vi "arranque.vi"   [LabVIEW 2016]
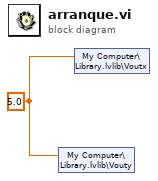
[diagram p0: block diagram]
diagram:
  w1 = 5.0
  n1 = shared-variable "My Computer\\Library.lvlib\\Vouty"(w1) -> ()  [unwired: 1 in, 1 out]
  n2 = shared-variable "My Computer\\Library.lvlib\\Voutx"(w1) -> ()  [unwired: 1 in, 1 out]
